vi "SLL DE AI Filter.vi"(8 "error in (no error)":errorcluster, 11 "Raw Data":dbl[][](array[numeric])) -> (0 "error out":errorcluster, 3 "Filtered Avg Data":dbl[][](array[numeric]))   [LabVIEW 2013]
uses:
  Controls/SLL DE DAQ Global Options.ctl
  Controls/SLL DE DAQ Global Elements.ctl
  <vilib>/Analysis/3filter.llb/Butterworth Filter (DBL).vi
  Instance           2 44Saved   AI Filter and Moving Average Data v1 .vi
  <vilib>/Analysis/NI_AALBase.lvlib
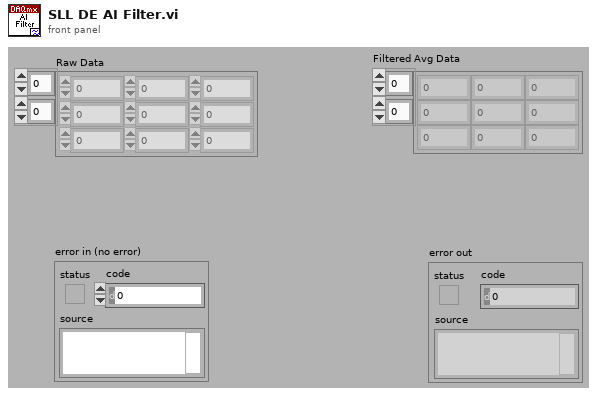
[diagram p1: front panel]
types:
  T1 = typedef "SLL DE DAQ Engine Parameters.ctl" = cluster{"Enable Engines":cluster{"AI Enable":bool, "AO Enable":bool, "DI Enable":bool, "DO Enable":bool}, "DAQ Control Type":cluster{"Analog Input":enum16{"Finite", "Continuous", "Driver"}, "Analog Output":enum16{"Finite", "Continuous", "Driver"}, "Digital Input":enum16{"Finite", "Continuous", "Driver"}, "Digital Output":enum16{"Finite", "Continuous", "Driver"}}, "DAQ Parameters":cluster{"AI Sampling Rate (Samples/Sec)":dbl, "MvgAVG Window Size (# of Points)":i32, "Enable Filter":bool, "Enable MvgAVG":bool, "Circular Buffer Size (Sec)":dbl, "AO Sampling Rate (Samples/Sec)":dbl, "Graph Update Rate (Samples/Sec)":dbl, "File Logging Rate (Samples/Sec)":i32}, "AO Safe Values":cluster{"Analog Outputs Name":T2, "Analog Outputs Safe Value":dbl}[], "DO Safe Values":cluster{"Digital Outputs Name":T3, "Digital Outputs Safe Value":bool}[], "DO Interconnected Lines":cluster{"First DO Line":string, "Second DO Line":string}[], "AI Channels Unit":cluster{"Channel Name":T4, "Channel Type":T5}[], "Units Information":cluster{"Channel Type":T5, "Unit Text":string, "Maximum":dbl, "Minmum":dbl, "Increments":dbl}[]}
  T2 = typedef "SLL DE List of Analog Outputs.ctl" = enum16{"None"}
  T3 = typedef "SLL DE List of Digital Outputs.ctl" = enum16{"STATION1_START TEST", "STATION1_STOP TEST", "STATION1_LIGHT1", "STATION1_LIGHT2", "STATION1_LIGHT3", "STATION2_START TEST", "STATION2_STOP TEST", "STATION2_LIGHT1", "STATION2_LIGHT2", "STATION2_LIGHT3", "STATION3_START TEST", "STATION3_STOP TEST", "STATION3_LIGHT1", "STATION3_LIGHT2", "STATION3_LIGHT3", "STATION4_START TEST", "STATION4_STOP TEST", "STATION4_LIGHT1", "STATION4_LIGHT2", "STATION4_LIGHT3"}
  T4 = typedef "SLL DE List of Analog Inputs.ctl" = enum16{"None"}
  T5 = typedef "SLL DE List of AI Channel Type.ctl" = enum16{"Pressure", "Flow", "Temperature", "Time Scale", "Voltage", "Current", "Frequency", "Sound", "Speed", "Torque", "Distance", "Channel Type 1", "Channel Type 2", "Channel Type 3"}
  T6 = enum32{"Lowpass", "Highpass", "Bandpass", "Bandstop"}
  T7 = typedef "SLL DE DAQ Global Elements.ctl" = enum16{"AI Error", "AO Error", "DI Error", "DO Error", "AI Restart", "DI Restart", "AI Running", "AO Running", "DI Running", "DO Running", "DAQ Exit?"}
  T8 = typedef "SLL DE DAQ Global Options.ctl" = enum16{"Init", "Write 1", "Read 1", "Write Array", "Read Array", "Clear"}
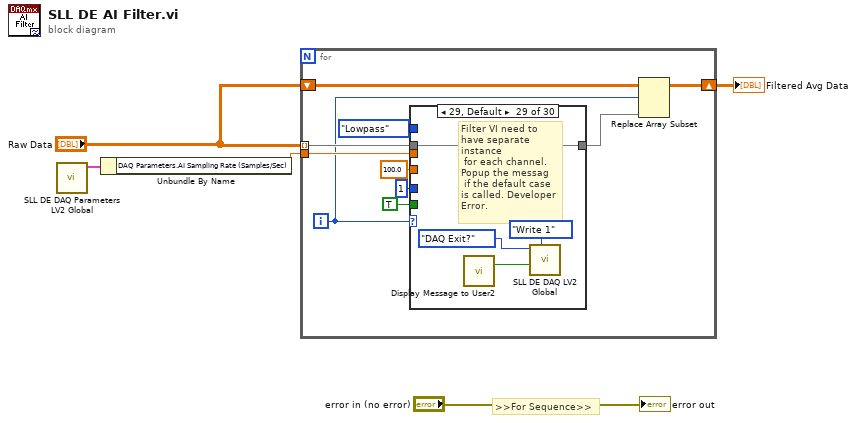
[diagram p0: block diagram]
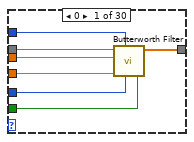
[diagram p2: hidden frame]
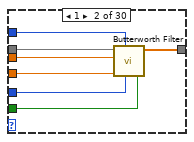
[diagram p3: hidden frame]
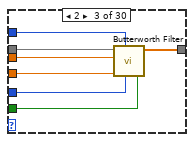
[diagram p4: hidden frame]
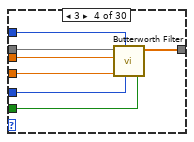
[diagram p5: hidden frame]
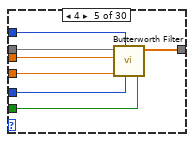
[diagram p6: hidden frame]
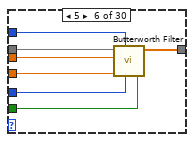
[diagram p7: hidden frame]
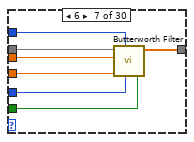
[diagram p8: hidden frame]
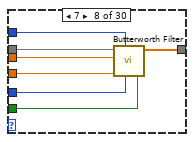
[diagram p9: hidden frame]
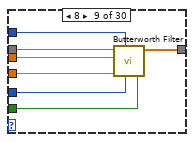
[diagram p10: hidden frame]
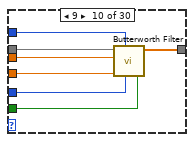
[diagram p11: hidden frame]
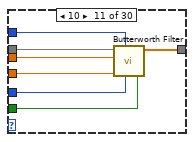
[diagram p12: hidden frame]
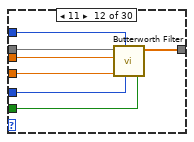
[diagram p13: hidden frame]
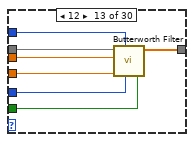
[diagram p14: hidden frame]
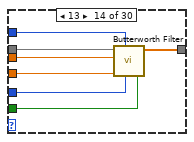
[diagram p15: hidden frame]
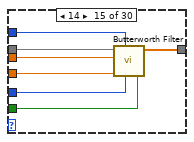
[diagram p16: hidden frame]
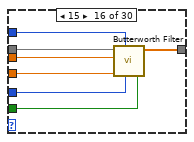
[diagram p17: hidden frame]
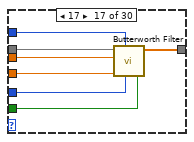
[diagram p18: hidden frame]
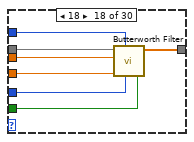
[diagram p19: hidden frame]
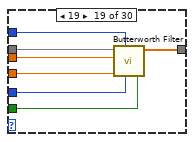
[diagram p20: hidden frame]
diagram:
  # ">>For Sequence>>"
  n1 = call "SLL DE DAQ Parameters LV2 Global.vi"() -> ("Global Info"=w4:T1)  [unwired: 10 in, 1 out]
  n2 = Unbundle By Name(w4) -> ("DAQ Parameters.AI Sampling Rate (Samples/Sec)"=w3:dbl)
  n3 = for {
    tunnel: "Raw Data" -> [w13] mode=indexing
    shift-right: [w15] -> w5
    shift-left: "Raw Data" -> [w14]
    tunnel: w3 -> [w12]
    i -> [w11]
    n4 = case shown="29, Default" w11 {
      tunnel: T6."Lowpass" ("filter type") -> [w22 w29 w36 w43 w50 w57 w64 w71 w78 w85 w92 w99 w106 w113 w120 w127 w134 w141 w148 w155 w162 w169 w176 w183 w190 w197 w204 w211 _ w222]
      tunnel: 1 ("order") -> [w21 w28 w35 w42 w49 w56 w63 w70 w77 w84 w91 w98 w105 w112 w119 w126 w133 w140 w147 w154 w161 w168 w175 w182 w189 w196 w203 w210 _ w221]
      tunnel: 100.0 ("low cutoff freq: fl") -> [w20 w27 w34 w41 w48 w55 w62 w69 w76 w83 w90 w97 w104 w111 w118 w125 w132 w139 w146 w153 w160 w167 w174 w181 w188 w195 w202 w209 _ w220]
      tunnel: w13 -> [w19 w26 w33 w40 w47 w54 w61 w68 w75 w82 w89 w96 w103 w110 w117 w124 w131 w138 w145 w152 w159 w166 w173 w180 w187 w194 w201 w208 w215 w219]
      tunnel: [w18 w25 w32 w39 w46 w53 w60 w67 w74 w81 w88 w95 w102 w109 w116 w123 w130 w137 w144 w151 w158 w165 w172 w179 w186 w193 w200 w207 w215 w218] -> w10
      tunnel: w12 -> [w17 w24 w31 w38 w45 w52 w59 w66 w73 w80 w87 w94 w101 w108 w115 w122 w129 w136 w143 w150 w157 w164 w171 w178 w185 w192 w199 w206 _ w217]
      tunnel: TRUE ("init/cont (init:F)") -> [w16 w23 w30 w37 w44 w51 w58 w65 w72 w79 w86 w93 w100 w107 w114 w121 w128 w135 w142 w149 w156 w163 w170 w177 w184 w191 w198 w205 _ w216]
      frame 0 {
        n5 = call-poly <vilib>:"Butterworth Filter.vi"("init/cont (init:F)"=w16, "order"=w21, "filter type"=w22, "low cutoff freq: fl"=w20, "sampling freq: fs"=w17, "X"=w19) -> ("Filtered X"=w18:dbl[])  [unwired: 2 in, 1 out]
      }
      frame 1 {
        n6 = call-poly <vilib>:"Butterworth Filter.vi"("init/cont (init:F)"=w23, "order"=w28, "filter type"=w29, "low cutoff freq: fl"=w27, "sampling freq: fs"=w24, "X"=w26) -> ("Filtered X"=w25:dbl[])  [unwired: 2 in, 1 out]
      }
      frame 2 {
        n7 = call-poly <vilib>:"Butterworth Filter.vi"("init/cont (init:F)"=w30, "order"=w35, "filter type"=w36, "low cutoff freq: fl"=w34, "sampling freq: fs"=w31, "X"=w33) -> ("Filtered X"=w32:dbl[])  [unwired: 2 in, 1 out]
      }
      frame 3 {
        n8 = call-poly <vilib>:"Butterworth Filter.vi"("init/cont (init:F)"=w37, "order"=w42, "filter type"=w43, "low cutoff freq: fl"=w41, "sampling freq: fs"=w38, "X"=w40) -> ("Filtered X"=w39:dbl[])  [unwired: 2 in, 1 out]
      }
      frame 4 {
        n9 = call-poly <vilib>:"Butterworth Filter.vi"("init/cont (init:F)"=w44, "order"=w49, "filter type"=w50, "low cutoff freq: fl"=w48, "sampling freq: fs"=w45, "X"=w47) -> ("Filtered X"=w46:dbl[])  [unwired: 2 in, 1 out]
      }
      frame 5 {
        n10 = call-poly <vilib>:"Butterworth Filter.vi"("init/cont (init:F)"=w51, "order"=w56, "filter type"=w57, "low cutoff freq: fl"=w55, "sampling freq: fs"=w52, "X"=w54) -> ("Filtered X"=w53:dbl[])  [unwired: 2 in, 1 out]
      }
      frame 6 {
        n11 = call-poly <vilib>:"Butterworth Filter.vi"("init/cont (init:F)"=w58, "order"=w63, "filter type"=w64, "low cutoff freq: fl"=w62, "sampling freq: fs"=w59, "X"=w61) -> ("Filtered X"=w60:dbl[])  [unwired: 2 in, 1 out]
      }
      frame 7 {
        n12 = call-poly <vilib>:"Butterworth Filter.vi"("init/cont (init:F)"=w65, "order"=w70, "filter type"=w71, "low cutoff freq: fl"=w69, "sampling freq: fs"=w66, "X"=w68) -> ("Filtered X"=w67:dbl[])  [unwired: 2 in, 1 out]
      }
      frame 8 {
        n13 = call-poly <vilib>:"Butterworth Filter.vi"("init/cont (init:F)"=w72, "order"=w77, "filter type"=w78, "low cutoff freq: fl"=w76, "sampling freq: fs"=w73, "X"=w75) -> ("Filtered X"=w74:dbl[])  [unwired: 2 in, 1 out]
      }
      frame 9 {
        n14 = call-poly <vilib>:"Butterworth Filter.vi"("init/cont (init:F)"=w79, "order"=w84, "filter type"=w85, "low cutoff freq: fl"=w83, "sampling freq: fs"=w80, "X"=w82) -> ("Filtered X"=w81:dbl[])  [unwired: 2 in, 1 out]
      }
      frame 10 {
        n15 = call-poly <vilib>:"Butterworth Filter.vi"("init/cont (init:F)"=w86, "order"=w91, "filter type"=w92, "low cutoff freq: fl"=w90, "sampling freq: fs"=w87, "X"=w89) -> ("Filtered X"=w88:dbl[])  [unwired: 2 in, 1 out]
      }
      frame 11 {
        n16 = call-poly <vilib>:"Butterworth Filter.vi"("init/cont (init:F)"=w93, "order"=w98, "filter type"=w99, "low cutoff freq: fl"=w97, "sampling freq: fs"=w94, "X"=w96) -> ("Filtered X"=w95:dbl[])  [unwired: 2 in, 1 out]
      }
      frame 12 {
        n17 = call-poly <vilib>:"Butterworth Filter.vi"("init/cont (init:F)"=w100, "order"=w105, "filter type"=w106, "low cutoff freq: fl"=w104, "sampling freq: fs"=w101, "X"=w103) -> ("Filtered X"=w102:dbl[])  [unwired: 2 in, 1 out]
      }
      frame 13 {
        n18 = call-poly <vilib>:"Butterworth Filter.vi"("init/cont (init:F)"=w107, "order"=w112, "filter type"=w113, "low cutoff freq: fl"=w111, "sampling freq: fs"=w108, "X"=w110) -> ("Filtered X"=w109:dbl[])  [unwired: 2 in, 1 out]
      }
      frame 14 {
        n19 = call-poly <vilib>:"Butterworth Filter.vi"("init/cont (init:F)"=w114, "order"=w119, "filter type"=w120, "low cutoff freq: fl"=w118, "sampling freq: fs"=w115, "X"=w117) -> ("Filtered X"=w116:dbl[])  [unwired: 2 in, 1 out]
      }
      frame 15 {
        n20 = call-poly <vilib>:"Butterworth Filter.vi"("init/cont (init:F)"=w121, "order"=w126, "filter type"=w127, "low cutoff freq: fl"=w125, "sampling freq: fs"=w122, "X"=w124) -> ("Filtered X"=w123:dbl[])  [unwired: 2 in, 1 out]
      }
      frame 17 {
        n21 = call-poly <vilib>:"Butterworth Filter.vi"("init/cont (init:F)"=w128, "order"=w133, "filter type"=w134, "low cutoff freq: fl"=w132, "sampling freq: fs"=w129, "X"=w131) -> ("Filtered X"=w130:dbl[])  [unwired: 2 in, 1 out]
      }
      frame 18 {
        n22 = call-poly <vilib>:"Butterworth Filter.vi"("init/cont (init:F)"=w135, "order"=w140, "filter type"=w141, "low cutoff freq: fl"=w139, "sampling freq: fs"=w136, "X"=w138) -> ("Filtered X"=w137:dbl[])  [unwired: 2 in, 1 out]
      }
      frame 19 {
        n23 = call-poly <vilib>:"Butterworth Filter.vi"("init/cont (init:F)"=w142, "order"=w147, "filter type"=w148, "low cutoff freq: fl"=w146, "sampling freq: fs"=w143, "X"=w145) -> ("Filtered X"=w144:dbl[])  [unwired: 2 in, 1 out]
      }
      frame 20 {
        n24 = call-poly <vilib>:"Butterworth Filter.vi"("init/cont (init:F)"=w149, "order"=w154, "filter type"=w155, "low cutoff freq: fl"=w153, "sampling freq: fs"=w150, "X"=w152) -> ("Filtered X"=w151:dbl[])  [unwired: 2 in, 1 out]
      }
      frame 21 {
        n25 = call-poly <vilib>:"Butterworth Filter.vi"("init/cont (init:F)"=w156, "order"=w161, "filter type"=w162, "low cutoff freq: fl"=w160, "sampling freq: fs"=w157, "X"=w159) -> ("Filtered X"=w158:dbl[])  [unwired: 2 in, 1 out]
      }
      frame 22 {
        n26 = call-poly <vilib>:"Butterworth Filter.vi"("init/cont (init:F)"=w163, "order"=w168, "filter type"=w169, "low cutoff freq: fl"=w167, "sampling freq: fs"=w164, "X"=w166) -> ("Filtered X"=w165:dbl[])  [unwired: 2 in, 1 out]
      }
      frame 23 {
        n27 = call-poly <vilib>:"Butterworth Filter.vi"("init/cont (init:F)"=w170, "order"=w175, "filter type"=w176, "low cutoff freq: fl"=w174, "sampling freq: fs"=w171, "X"=w173) -> ("Filtered X"=w172:dbl[])  [unwired: 2 in, 1 out]
      }
      frame 24 {
        n28 = call-poly <vilib>:"Butterworth Filter.vi"("init/cont (init:F)"=w177, "order"=w182, "filter type"=w183, "low cutoff freq: fl"=w181, "sampling freq: fs"=w178, "X"=w180) -> ("Filtered X"=w179:dbl[])  [unwired: 2 in, 1 out]
      }
      frame 25 {
        n29 = call-poly <vilib>:"Butterworth Filter.vi"("init/cont (init:F)"=w184, "order"=w189, "filter type"=w190, "low cutoff freq: fl"=w188, "sampling freq: fs"=w185, "X"=w187) -> ("Filtered X"=w186:dbl[])  [unwired: 2 in, 1 out]
      }
      frame 26 {
        n30 = call-poly <vilib>:"Butterworth Filter.vi"("init/cont (init:F)"=w191, "order"=w196, "filter type"=w197, "low cutoff freq: fl"=w195, "sampling freq: fs"=w192, "X"=w194) -> ("Filtered X"=w193:dbl[])  [unwired: 2 in, 1 out]
      }
      frame 27 {
        n31 = call-poly <vilib>:"Butterworth Filter.vi"("init/cont (init:F)"=w198, "order"=w203, "filter type"=w204, "low cutoff freq: fl"=w202, "sampling freq: fs"=w199, "X"=w201) -> ("Filtered X"=w200:dbl[])  [unwired: 2 in, 1 out]
      }
      frame 28 {
        n32 = call-poly <vilib>:"Butterworth Filter.vi"("init/cont (init:F)"=w205, "order"=w210, "filter type"=w211, "low cutoff freq: fl"=w209, "sampling freq: fs"=w206, "X"=w208) -> ("Filtered X"=w207:dbl[])  [unwired: 2 in, 1 out]
      }
      frame 29, Default {
        # "Filter VI need to have separate instance\n for each channel. Popup the messag\n if the default case is called. Developer Error."
        n33 = call "Display Message to User2"() -> ("Exit"=w213:bool)  [unwired: 10 in, 1 out]
        n34 = call "SLL DE DAQ LV2 Global.vi"("Option"=SLL_DE_DAQ_Global_Options."Write 1", "Status In"=w213, "Element"=SLL_DE_DAQ_Global_Elements."DAQ Exit?") -> ()  [unwired: 6 in, 3 out]
      }
      frame 16 {
        n35 = call-poly <vilib>:"Butterworth Filter.vi"("init/cont (init:F)"=w216, "order"=w221, "filter type"=w222, "low cutoff freq: fl"=w220, "sampling freq: fs"=w217, "X"=w219) -> ("Filtered X"=w218:dbl[])  [unwired: 2 in, 1 out]
      }
    }
    n36 = Replace Array Subset(array=w14, new element=w10, index (row)=w11) -> (w15:dbl[][])  [unwired: 1 in]
  }
  "Filtered Avg Data" <- w5
  "error out" <- "error in (no error)"
